vi "NXTMMX-DM.old2.vi"(0 "Input of Motor Multiplexer":T4={"NXTMMX Address"=6, "Which Motor"=0, "Operation"=0, "Next Action"=0, "Position"=0, "Direction"=FALSE, "Power"=100, "Durartion"=0, "Wait for Completion"=FALSE, "Relative"=FALSE, "PID"={"Write PID"=FALSE, "PKp"=100, "PKi"=100, "PKd"=100, "SKp "=100, "SKi"=100, "SKd"=100, "passcount"=0, "tolerance"=0}} {"Next Action" items=["Float", "Brake"]; "Operation" items=["Run Unlimited", "Run Seconds", "Run Tachometer"]; "Which Motor" items=["Motor 1", "Motor 2", "Both Motors"]; "NXTMMX Address" min=2 max=254 step=2 format="%x"}, 2 "NXT":T2={"Hardware"="NXT", "Flattened String"=""}, 3 "Input Port":T3 items=["Port 1", "Port 2", "Port 3", "Port 4"]) -> (1 "Output of Motor Multiplexer":T1, 4 "NXT dup":T2={"Hardware"="NXT", "Flattened String"=""})   [LabVIEW 2010]
uses:
  <vilib>/NXT/Block Support/NXT_InputPort.ctl
  <vilib>/NXT/Subs/LVHSConnector.ctl
  <vilib>/NXT/Block Support/HWPage.SensorType.ctl
  <vilib>/NXT/Block Support/HWPage.SensorMode.ctl
  <vilib>/NXT/Dual Mode Library/Waits/Wait_Num(msec).vi
panel:
  out "Address":i32
  # "mindsensors.com\nCopyright (c) 2009 by mindsensors.com\nEmail: info (<at>) mindsensors (<dot>) com\n\nThis program is free software. You can redistribute it and/or modify\nit under the terms of the GNU General Public License as published by\nthe Free Software Foundation; version 3 of the License.\nRead the license at: http://www.gnu.org/licenses/gpl.txt"
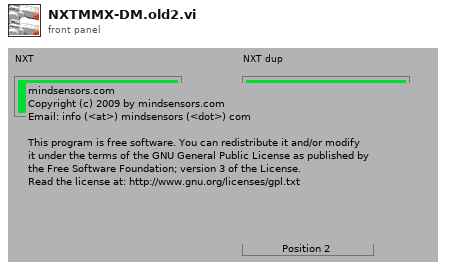
[diagram p1: front panel]
types:
  T1 = cluster{"Milivolts":u16, "Position 1":i32, "Position 2":i32, "Motor battery Voltage":dbl}
  T2 = typedef "LVHSConnector.ctl" = cluster{"Hardware":string, "Flattened String":string}
  T3 = typedef "NXT_InputPort.ctl" = u8
  T4 = cluster{"NXTMMX Address":u8, "Which Motor":u8, "Operation":u8, "Next Action":u8, "Position":i32, "Direction":bool, "Power":i8, "Durartion":u8, "Wait for Completion":bool, "Relative":bool, "PID":cluster{"Write PID":bool, "PKp":u16, "PKi":u16, "PKd":u16, "SKp ":u16, "SKi":u16, "SKd":u16, "passcount":u8, "tolerance":u8}}
  T5 = typedef "HWPage.SensorType.ctl" = u8
  T6 = typedef "HWPage.SensorMode.ctl" = u8
  T7 = cluster{"Write PID":bool, "PKp":u16, "PKi":u16, "PKd":u16, "SKp ":u16, "SKi":u16, "SKd":u16, "passcount":u8, "tolerance":u8}
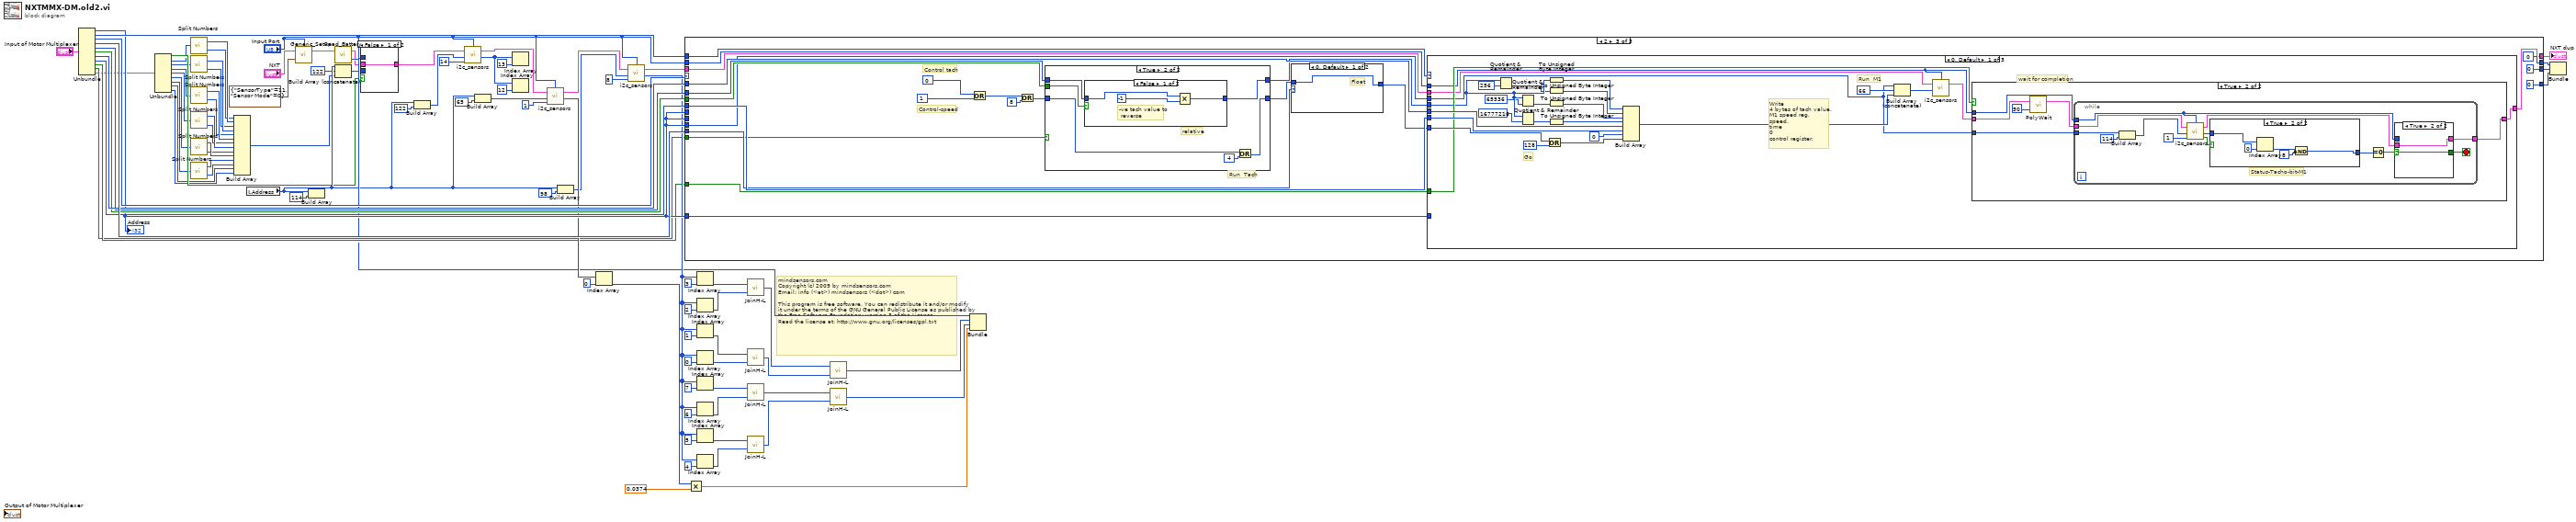
[diagram p0: block diagram]
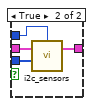
[diagram p2: hidden frame]
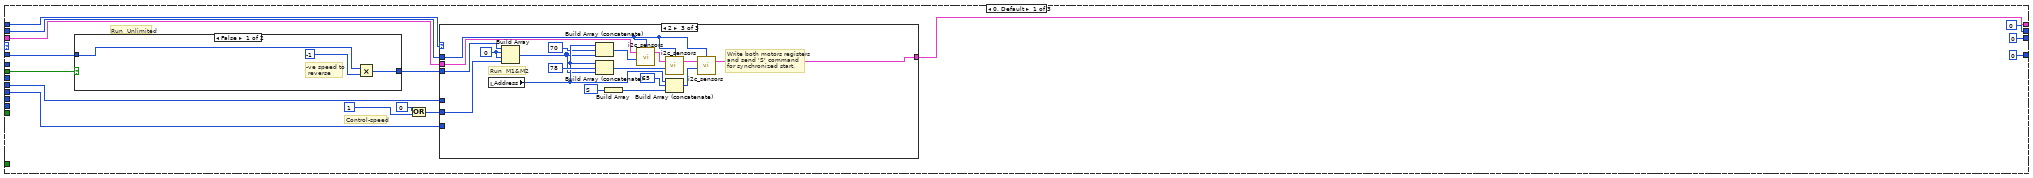
[diagram p3: hidden frame]
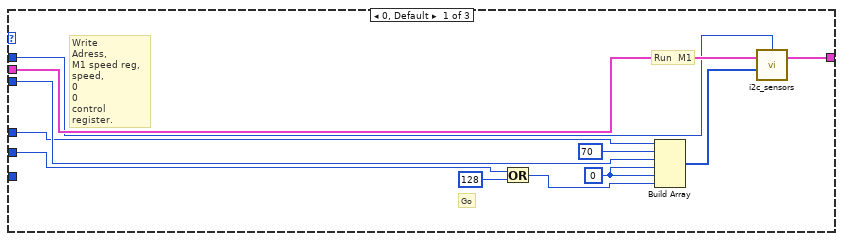
[diagram p4: hidden frame]
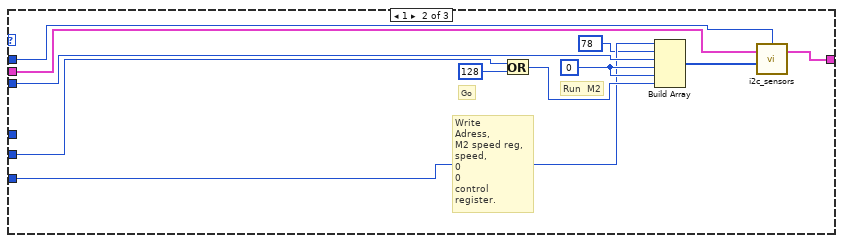
[diagram p5: hidden frame]
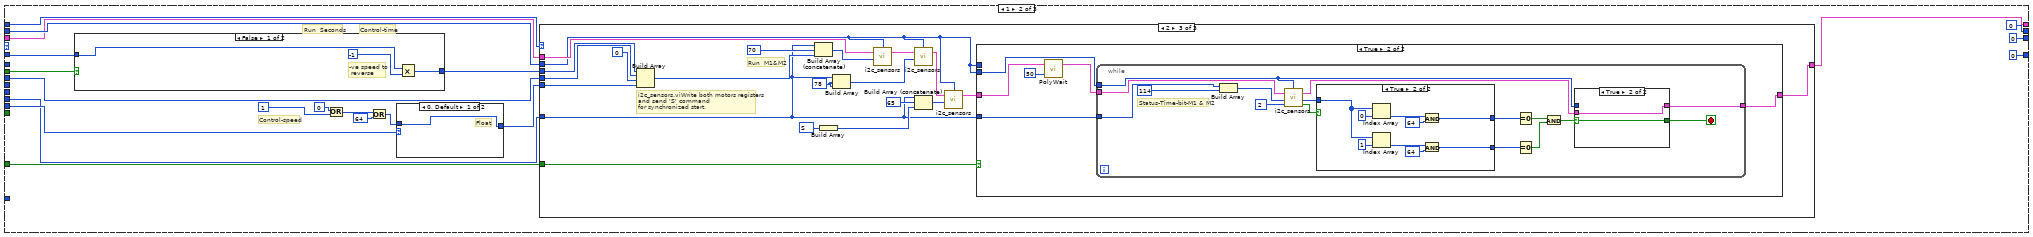
[diagram p7: hidden frame]
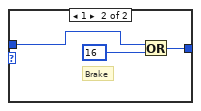
[diagram p8: hidden frame]
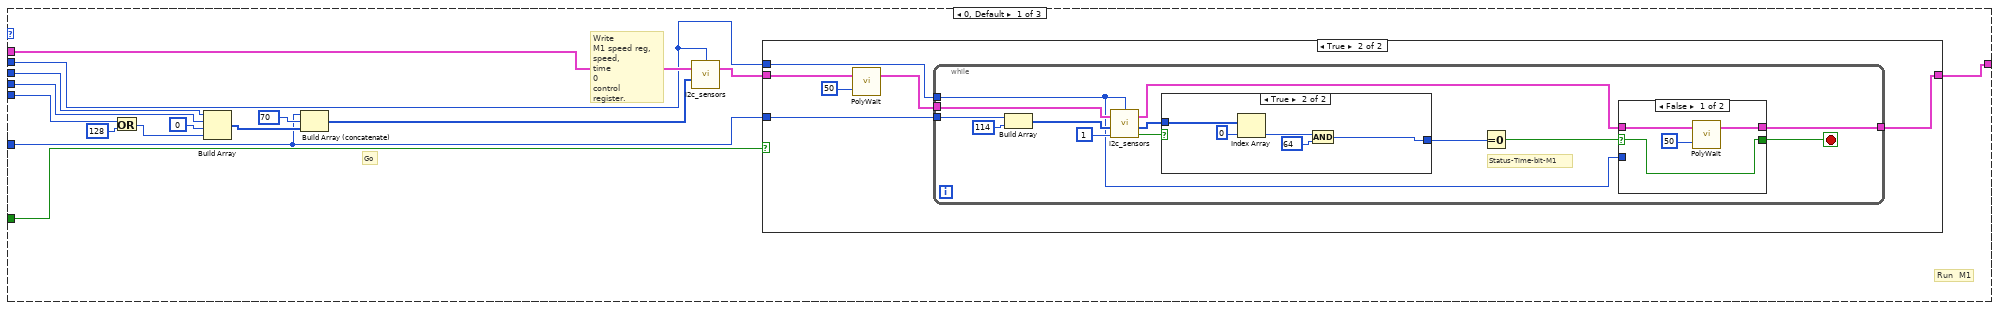
[diagram p9: hidden frame]
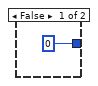
[diagram p12: hidden frame]
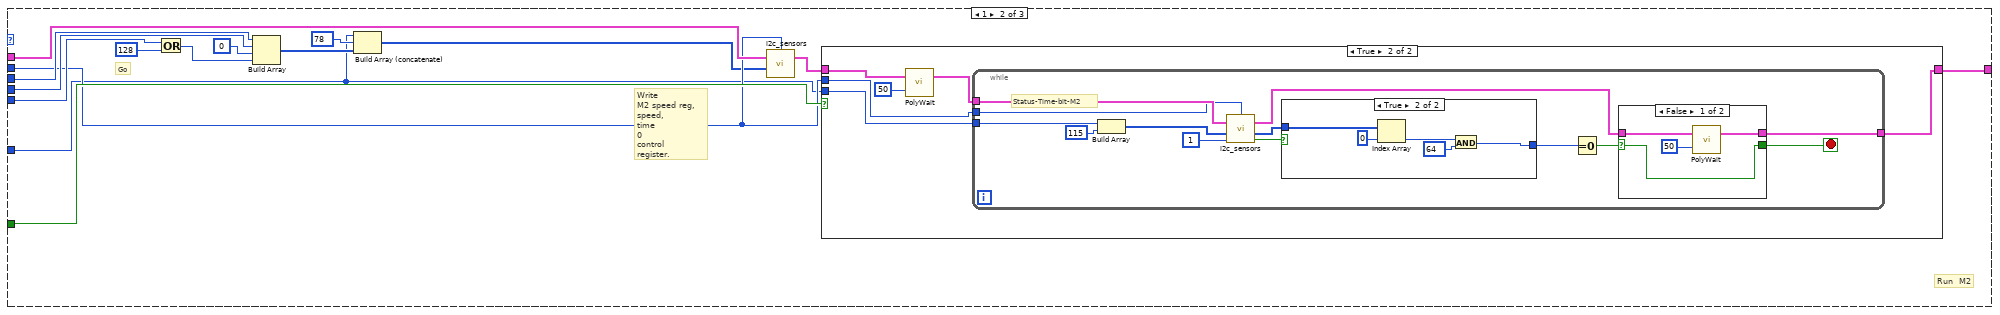
[diagram p13: hidden frame]
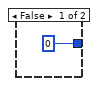
[diagram p16: hidden frame]
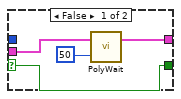
[diagram p18: hidden frame]
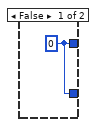
[diagram p19: hidden frame]
diagram:
  # "mindsensors.com\nCopyright (c) 2009 by mindsensors.com\nEmail: info (<at>) mindsensors (<dot>) com\n\nThis program is free software. You can redistribute it and/or modify\nit under the terms of the GNU General Public License as published by\nthe Free Software Foundation; version 3 of the License.\nRead the license at: http://www.gnu.org/licenses/gpl.txt"
  n1 = Unbundle("Input of Motor Multiplexer") -> ("NXTMMX Address"=w84:u8, "Which Motor"=w86:u8, "Operation"=w91:u8, "Next Action"=w90:u8, "Position"=w88:i32, "Direction"=w87:bool, "Power"=w89:i8, "Durartion"=w85:u8, "Wait for Completion"=w50:bool, "Relative"=w49:bool, "PID"=w33:T7)
  "Address" <- w84
  n2 = Unbundle(w33) -> ("Write PID"=w36:bool, "PKp"=w18:u16, "PKi"=w15:u16, "PKd"=w10:u16, "SKp"=w7:u16, "SKi"=w4:u16, "SKd"=w3:u16, "passcount"=w35:u8, "tolerance"=w34:u8)
  n3 = call <vilib>:"Split Numbers.vi"("(hi.lo)"=w18) -> ("low"=w16:u8, "hi"=w17:u8)
  n4 = call <vilib>:"Split Numbers.vi"("(hi.lo)"=w15) -> ("low"=w13:u8, "hi"=w14:u8)
  n5 = call <vilib>:"Split Numbers.vi"("(hi.lo)"=w10) -> ("low"=w11:u8, "hi"=w12:u8)
  n6 = call <vilib>:"Split Numbers.vi"("(hi.lo)"=w7) -> ("low"=w8:u8, "hi"=w9:u8)
  n7 = call <vilib>:"Split Numbers.vi"("(hi.lo)"=w4) -> ("low"=w5:u8, "hi"=w6:u8)
  n8 = call <vilib>:"Split Numbers.vi"("(hi.lo)"=w3) -> ("low"=w1:u8, "hi"=w2:u8)
  n9 = Build Array(w16, w17, w13, w14, w11, w12, w8, w9, w5, w6, w2, w1, w35, w34) -> (w41:u8[])
  n10 = local read "Address"() -> (w43:i32)
  n11 = call <vilib>:"Generic_Setup.vi"("Sensor Setup"=cluster{"SensorType":T5, "Sensor Mode":T6} {"SensorType"=11, "Sensor Mode"=0}, "NXT"="NXT", "Port"="Input Port") -> ("NXT"=w82:T2)  [unwired: 1 out]
  n12 = Build Array(w43, u8 114 ("Reg Address")) -> ()  [unwired: 1 out]
  n13 = call <vilib>:"Read_Battery.vi"("NXT"=w82) -> ("millivolts"=w48:i32, "NXT"=w38:T2)  [unwired: 2 in]
  n14 = Build Array (concatenate)(w43, u8 122 ("Reg Address"), w41) -> (w40:i32[])
  n15 = case shown="False" w36 {
    tunnel: w40 -> [_ w97]
    tunnel: "Input Port" -> [_ w96]
    tunnel: w38 -> [w93 w95]
    tunnel: [w93 w94] -> w37
    frame False {
    }
    frame True {
      n16 = call <vilib>:"i2c_sensors.vi"("Bytes to Write"=w97, "NXT"=w95, "Port"=w96) -> ("NXT"=w94:T2)  [unwired: 2 in, 2 out]
    }
  }
  n17 = Build Array(w43, u8 122 ("Reg Address")) -> (w67:i32[])
  n18 = call <vilib>:"i2c_sensors.vi"("Return Length"=u8 14 ("bytes to read"), "Bytes to Write"=w67, "NXT"=w37, "Port"="Input Port") -> ("Bytes read"=w65:u8[], "NXT"=w60:T2)  [unwired: 1 in, 1 out]
  n19 = Build Array(w43, u8 65 ("Reg Address")) -> (w62:i32[])
  n20 = Index Array(array=w65, index=13) -> ()  [unwired: 1 out]
  n21 = Index Array(array=w65, index=12) -> ()  [unwired: 1 out]
  n22 = call <vilib>:"i2c_sensors.vi"("Return Length"=u8 1 ("bytes to read"), "Bytes to Write"=w62, "NXT"=w60, "Port"="Input Port") -> ("Bytes read"=w61:u8[], "NXT"=w55:T2)  [unwired: 1 in, 1 out]
  n23 = Build Array(w43, u8 98 ("Reg Address")) -> (w59:i32[])
  n24 = Index Array(array=w61, index=0) -> (element=w70:u8)
  n25 = call <vilib>:"i2c_sensors.vi"("Return Length"=u8 8 ("bytes to read"), "Bytes to Write"=w59, "NXT"=w55, "Port"="Input Port") -> ("Bytes read"=w56:u8[], "NXT"=w52:T2)  [unwired: 1 in, 1 out]
  n26 = case shown="2" w91 {
    tunnel: w87 -> [w110 w174 w360]
    tunnel: w89 -> [w109 w173 w350]
    tunnel: w86 -> [w108 w172 w359]
    tunnel: "Input Port" -> [w106 w170 w358]
    tunnel: w85 -> [_ w167 w355]
    tunnel: w90 -> [_ w166 w354]
    tunnel: w88 -> [_ _ w351]
    tunnel: w50 -> [_ w163 w352]
    tunnel: w49 -> [_ _ w348]
    tunnel: [0 0 0] -> w47
    tunnel: [u32 0 ("Out") u32 0 ("Out") u32 0 ("Out")] -> w46
    tunnel: [u16 0 u16 0 u16 0] -> w45
    tunnel: w52 -> [w101 w159 w341]
    tunnel: [w100 w158 w342] -> w44
    tunnel: w84 -> [_ w157 w340]
    tunnel: w84 -> [w99 _ _]
    tunnel: w84 -> [_ _ w339]
    tunnel: w84 -> [w98 _ _]
    frame 0, Default {
      # "Control-speed"
      # "Run  Unlimited"
      n27 = case shown="False" w110 {
        tunnel: w109 -> [w155 w156]
        tunnel: [w153 w156] -> w107
        frame False {
          # "-ve speed to\n reverse"
          n28 = Multiply(x=w155, y=i8 -1) -> (x*y=w153:i8)
        }
        frame True {
        }
      }
      n29 = Or(x=0, y=1) -> (x .or. y?=w105:i32)
      n30 = case shown="2" w108 {
        tunnel: w105 -> [w122 w133 w149]
        tunnel: w107 -> [w121 w132 w152]
        tunnel: w106 -> [w116 w129 w144]
        tunnel: w101 -> [w118 w128 w148]
        tunnel: [w117 w127 w139] -> w100
        tunnel: w99 -> [w115 _ _]
        tunnel: w98 -> [_ w126 _]
        frame 0, Default {
          w120 = 0
          # "Go"
          # "Run  M1"
          # "Write \nAdress,\nM1 speed reg,\nspeed,\n0\n0\ncontrol register."
          n31 = Or(x=w122, y=128) -> (x .or. y?=w119:i32)
          n32 = Build Array(w115, 70, w121, w120, w120, w119) -> (w113:i32[])
          n33 = call <vilib>:"i2c_sensors.vi"("Bytes to Write"=w113, "NXT"=w118, "Port"=w116) -> ("NXT"=w117:T2)  [unwired: 2 in, 2 out]
        }
        frame 1 {
          w131 = 0
          # "Go"
          # "Run  M2"
          # "Write\nAdress, \nM2 speed reg,\nspeed,\n0\n0\ncontrol register."
          n34 = Or(x=w133, y=128) -> (x .or. y?=w130:i32)
          n35 = Build Array(w126, 78, w132, w131, w131, w130) -> (w124:i32[])
          n36 = call <vilib>:"i2c_sensors.vi"("Bytes to Write"=w124, "NXT"=w128, "Port"=w129) -> ("NXT"=w127:T2)  [unwired: 2 in, 2 out]
        }
        frame 2 {
          w150 = u16 83 items=["S"=83]
          w151 = 0
          # "Write both motors registers\nand send 'S' command \nfor synchronized start."
          # "Run  M1&M2"
          n37 = local read "Address"() -> (w138:i32)
          n38 = Build Array(w152, w151, w151, w149) -> (w135:i32[])
          n39 = Build Array (concatenate)(w138, 70, w135) -> (w136:i32[])
          n40 = Build Array (concatenate)(w138, 78, w135) -> (w146:i32[])
          n41 = Build Array(w150) -> (w142:u16[])
          n42 = call <vilib>:"i2c_sensors.vi"("Bytes to Write"=w136, "NXT"=w148, "Port"=w144) -> ("NXT"=w145:T2)  [unwired: 2 in, 2 out]
          n43 = call <vilib>:"i2c_sensors.vi"("Bytes to Write"=w146, "NXT"=w145, "Port"=w144) -> ("NXT"=w143:T2)  [unwired: 2 in, 2 out]
          n44 = Build Array (concatenate)(w138, 65, w142) -> (w140:i32[])
          n45 = call <vilib>:"i2c_sensors.vi"("Bytes to Write"=w140, "NXT"=w143, "Port"=w144) -> ("NXT"=w139:T2)  [unwired: 2 in, 2 out]
        }
      }
    }
    frame 1 {
      # "Control-time"
      # "Control-speed"
      # "Run  Seconds"
      n46 = case shown="False" w174 {
        tunnel: w173 -> [w337 w338]
        tunnel: [w335 w338] -> w171
        frame False {
          # "-ve speed to\n reverse"
          n47 = Multiply(x=w337, y=i8 -1) -> (x*y=w335:i8)
        }
        frame True {
        }
      }
      n48 = Or(x=0, y=1) -> (x .or. y?=w168:i32)
      n49 = Or(x=w168, y=64) -> (x .or. y?=w165:i32)
      n50 = case shown="0, Default" w166 {
        tunnel: w165 -> [w177 w179]
        tunnel: [w177 w180] -> w164
        frame 0, Default {
          # "Float"
        }
        frame 1 {
          # "Brake"
          n51 = Or(x=w179, y=16) -> (x .or. y?=w180:i32)
        }
      }
      n52 = case shown="2" w172 {
        tunnel: w164 -> [w194 w241 w292]
        tunnel: w171 -> [w193 w240 w295]
        tunnel: w170 -> [w183 w232 w277]
        tunnel: w167 -> [w190 w237 w291]
        tunnel: w163 -> [w189 w236 w290]
        tunnel: w159 -> [w187 w235 w286]
        tunnel: [w182 w229 w276] -> w158
        tunnel: w157 -> [w181 w228 w275]
        frame 0, Default {
          # "Go"
          # "Run  M1"
          # "Write \nM1 speed reg,\nspeed,\ntime\n0\ncontrol register."
          n53 = Or(x=w194, y=128) -> (x .or. y?=w191:i32)
          n54 = Build Array(w193, w190, 0, w191) -> (w184:i32[])
          n55 = Build Array (concatenate)(w181, 70, w184) -> (w186:i32[])
          n56 = call <vilib>:"i2c_sensors.vi"("Bytes to Write"=w186, "NXT"=w187, "Port"=w183) -> ("NXT"=w188:T2)  [unwired: 2 in, 2 out]
          n57 = case shown="True" w189 {
            tunnel: w183 -> [_ w202]
            tunnel: w188 -> [w196 w200]
            tunnel: [w196 w198] -> w182
            tunnel: w181 -> [_ w197]
            frame False {
            }
            frame True {
              n58 = call-poly <vilib>:"PolyWait.vi"("Time (100 msec)"=u16 50 ("Delay ms"), "NXT"=w200) -> ("NXT"=w199:T2)  [unwired: 2 in]
              n59 = while {
                tunnel: w202 -> [w206]
                tunnel: w199 -> [w211]
                tunnel: [w210] -> w198
                tunnel: w197 -> [w204]
                stop <- w214 stop-if-true
                # "Status-Time-bit-M1"
                n60 = Build Array(w204, 114) -> (w207:i32[])
                n61 = call <vilib>:"i2c_sensors.vi"("Return Length"=1, "Bytes to Write"=w207, "NXT"=w211, "Port"=w206) -> ("Success?"=w203:bool, "Bytes read"=w209:u8[], "NXT"=w212:T2)  [unwired: 1 in]
                n62 = case shown="True" w203 {
                  tunnel: w209 -> [_ w227]
                  tunnel: [u8 0 w223] -> w215
                  frame False {
                  }
                  frame True {
                    n63 = Index Array(array=w227, index=0) -> (element=w224:u8)
                    n64 = And(x=w224, y=u8 64) -> (x .and. y?=w223:u8)
                  }
                }
                n65 = Equal To 0?(x=w215) -> (x = 0?=w213:bool)
                n66 = case shown="False" w213 {
                  selector: w213 -> [w219 w221]
                  tunnel: w206 -> [_ _]
                  tunnel: [w219 w221] -> w214
                  tunnel: w212 -> [w217 w220]
                  tunnel: [w216 w220] -> w210
                  frame False {
                    n67 = call-poly <vilib>:"PolyWait.vi"("Time (100 msec)"=u16 50 ("Delay ms"), "NXT"=w217) -> ("NXT"=w216:T2)  [unwired: 2 in]
                  }
                  frame True {
                  }
                }
              }
            }
          }
        }
        frame 1 {
          # "Go"
          # "Run  M2"
          # "Write \nM2 speed reg,\nspeed,\ntime\n0\ncontrol register."
          n68 = Or(x=w241, y=128) -> (x .or. y?=w238:i32)
          n69 = Build Array(w240, w237, 0, w238) -> (w233:i32[])
          n70 = Build Array (concatenate)(w228, 78, w233) -> (w231:i32[])
          n71 = call <vilib>:"i2c_sensors.vi"("Bytes to Write"=w231, "NXT"=w235, "Port"=w232) -> ("NXT"=w230:T2)  [unwired: 2 in, 2 out]
          n72 = case shown="True" w236 {
            tunnel: w232 -> [_ w249]
            tunnel: w230 -> [w243 w247]
            tunnel: [w243 w245] -> w229
            tunnel: w228 -> [_ w244]
            frame False {
            }
            frame True {
              n73 = call-poly <vilib>:"PolyWait.vi"("Time (100 msec)"=u16 50 ("Delay ms"), "NXT"=w247) -> ("NXT"=w246:T2)  [unwired: 2 in]
              n74 = while {
                tunnel: w249 -> [w256]
                tunnel: w246 -> [w257]
                tunnel: [w259] -> w245
                tunnel: w244 -> [w251]
                stop <- w261 stop-if-true
                # "Status-Time-bit-M2"
                n75 = Build Array(w251, 115) -> (w253:i32[])
                n76 = call <vilib>:"i2c_sensors.vi"("Return Length"=1, "Bytes to Write"=w253, "NXT"=w257, "Port"=w256) -> ("Success?"=w250:bool, "Bytes read"=w252:u8[], "NXT"=w258:T2)  [unwired: 1 in]
                n77 = case shown="True" w250 {
                  tunnel: w252 -> [_ w274]
                  tunnel: [u8 0 w270] -> w262
                  frame False {
                  }
                  frame True {
                    n78 = Index Array(array=w274, index=0) -> (element=w271:u8)
                    n79 = And(x=w271, y=u8 64) -> (x .and. y?=w270:u8)
                  }
                }
                n80 = Equal To 0?(x=w262) -> (x = 0?=w260:bool)
                n81 = case shown="False" w260 {
                  selector: w260 -> [w266 w268]
                  tunnel: [w266 w268] -> w261
                  tunnel: [w264 w267] -> w259
                  tunnel: w258 -> [w263 w267]
                  frame False {
                    n82 = call-poly <vilib>:"PolyWait.vi"("Time (100 msec)"=u16 50 ("Delay ms"), "NXT"=w263) -> ("NXT"=w264:T2)  [unwired: 2 in]
                  }
                  frame True {
                  }
                }
              }
            }
          }
        }
        frame 2 {
          w293 = u16 83 items=["S"=83]
          w285 = 78
          # "i2c_sensors.viWrite both motors registers\nand send 'S' command \nfor synchronized start."
          # "Run  M1&M2"
          n83 = Build Array(w295, w291, 0, w292) -> (w288:i32[])
          n84 = Build Array (concatenate)(w275, 70, w288) -> (w287:i32[])
          n85 = Build Array(w293) -> (w283:u16[])
          n86 = Build Array(w275, w285, w285) -> (w280:i32[])
          n87 = call <vilib>:"i2c_sensors.vi"("Bytes to Write"=w287, "NXT"=w286, "Port"=w277) -> ("NXT"=w281:T2)  [unwired: 2 in, 2 out]
          n88 = call <vilib>:"i2c_sensors.vi"("Bytes to Write"=w280, "NXT"=w281, "Port"=w277) -> ("NXT"=w282:T2)  [unwired: 2 in, 2 out]
          n89 = Build Array (concatenate)(w275, 65, w283) -> (w279:i32[])
          n90 = call <vilib>:"i2c_sensors.vi"("Bytes to Write"=w279, "NXT"=w282, "Port"=w277) -> ("NXT"=w278:T2)  [unwired: 2 in, 2 out]
          n91 = case shown="True" w290 {
            tunnel: w277 -> [_ _]
            tunnel: w278 -> [w296 w301]
            tunnel: w277 -> [_ w299]
            tunnel: [w296 w298] -> w276
            tunnel: w275 -> [_ w297]
            frame False {
            }
            frame True {
              n92 = call-poly <vilib>:"PolyWait.vi"("Time (100 msec)"=u16 50 ("Delay ms"), "NXT"=w301) -> ("NXT"=w300:T2)  [unwired: 2 in]
              n93 = while {
                tunnel: w300 -> [w306]
                tunnel: w299 -> [w309]
                tunnel: [w305] -> w298
                tunnel: w297 -> [w304]
                stop <- w313 stop-if-true
                # "Status-Time-bit-M1 & M2"
                n94 = Build Array(w304, 114) -> (w310:i32[])
                n95 = call <vilib>:"i2c_sensors.vi"("Return Length"=2, "Bytes to Write"=w310, "NXT"=w306, "Port"=w309) -> ("Success?"=w303:bool, "Bytes read"=w308:u8[], "NXT"=w307:T2)  [unwired: 1 in]
                n96 = case shown="True" w303 {
                  tunnel: w308 -> [_ w333]
                  tunnel: [w325 w326] -> w318
                  tunnel: [w325 w328] -> w317
                  frame False {
                    w325 = u8 0
                  }
                  frame True {
                    n97 = Index Array(array=w333, index=0) -> (element=w329:u8)
                    n98 = Index Array(array=w333, index=1) -> (element=w327:u8)
                    n99 = And(x=w329, y=u8 64) -> (x .and. y?=w328:u8)
                    n100 = And(x=w327, y=u8 64) -> (x .and. y?=w326:u8)
                  }
                }
                n101 = Equal To 0?(x=w317) -> (x = 0?=w316:bool)
                n102 = Equal To 0?(x=w318) -> (x = 0?=w315:bool)
                n103 = And(x=w316, y=w315) -> (x .and. y?=w314:bool)
                n104 = case shown="True" w314 {
                  selector: w314 -> [w322 w324]
                  tunnel: w309 -> [_ _]
                  tunnel: [w322 w324] -> w313
                  tunnel: w307 -> [w320 w323]
                  tunnel: [w319 w323] -> w305
                  frame False {
                    n105 = call-poly <vilib>:"PolyWait.vi"("Time (100 msec)"=u16 50 ("Delay ms"), "NXT"=w320) -> ("NXT"=w319:T2)  [unwired: 2 in]
                  }
                  frame True {
                  }
                }
              }
            }
          }
        }
      }
    }
    frame 2 {
      # "Run  Tach"
      # "Control tach"
      # "Control-speed"
      n106 = Or(x=0, y=1) -> (x .or. y?=w356:i32)
      n107 = Or(x=w356, y=8) -> (x .or. y?=w347:i32)
      n108 = case shown="True" w348 {
        tunnel: w360 -> [_ w370]
        tunnel: w351 -> [w364 w369]
        tunnel: [w364 w368] -> w349
        tunnel: w347 -> [w363 w367]
        tunnel: [w363 w365] -> w346
        frame False {
          # "absolute\nignore the direction"
        }
        frame True {
          # "relative"
          n109 = case shown="False" w370 {
            tunnel: w369 -> [w373 w374]
            tunnel: [w371 w374] -> w368
            frame False {
              # "-ve tach value to\n reverse"
              n110 = Multiply(x=w373, y=i8 -1) -> (x*y=w371:i32)
            }
            frame True {
            }
          }
          n111 = Or(x=w367, y=4) -> (x .or. y?=w365:i32)
        }
      }
      n112 = case shown="0, Default" w354 {
        tunnel: [w375 w378] -> w353
        tunnel: w346 -> [w375 w376]
        frame 0, Default {
          # "Float"
        }
        frame 1 {
          # "Brake"
          n113 = Or(x=w376, y=16) -> (x .or. y?=w378:i32)
        }
      }
      n114 = case shown="0, Default" w359 {
        tunnel: w353 -> [w403 w461 w524]
        tunnel: w358 -> [w385 w442 w496]
        tunnel: w355 -> [w399 w457 w523]
        tunnel: w352 -> [w398 w456 w522]
        tunnel: w350 -> [w402 w460 w521]
        tunnel: w349 -> [w396 w449 w514]
        tunnel: [w379 w437 w509] -> w342
        tunnel: w341 -> [w382 w440 w508]
        tunnel: w340 -> [w380 _ _]
        tunnel: w339 -> [_ w438 _]
        frame 0, Default {
          # "wait for completion"
          # "Go"
          # "Run  M1"
          # "Write\n4 bytes of tach value. \nM1 speed reg,\nspeed,\ntime\n0\ncontrol register."
          n115 = Quotient & Remainder(x=w396, y=u32 256) -> (floor(x/y)=w392:u32)  [unwired: 1 out]
          n116 = Quotient & Remainder(x=w396, y=u32 65536) -> (floor(x/y)=w390:u32)  [unwired: 1 out]
          n117 = Quotient & Remainder(x=w396, y=u32 16777216) -> (floor(x/y)=w387:u32)  [unwired: 1 out]
          n118 = Or(x=w403, y=128) -> (x .or. y?=w400:i32)
          n119 = To Unsigned Byte Integer(number=w396) -> (unsigned 8bit integer=w397:u8)
          n120 = To Unsigned Byte Integer(number=w392) -> (unsigned 8bit integer=w391:u8)
          n121 = To Unsigned Byte Integer(number=w390) -> (unsigned 8bit integer=w389:u8)
          n122 = To Unsigned Byte Integer(number=w387) -> (unsigned 8bit integer=w388:u8)
          n123 = Build Array(w397, w391, w389, w388, w402, w399, 0, w400) -> (w386:i32[])
          n124 = Build Array (concatenate)(w380, 66, w386) -> (w383:i32[])
          n125 = call <vilib>:"i2c_sensors.vi"("Bytes to Write"=w383, "NXT"=w382, "Port"=w385) -> ("NXT"=w381:T2)  [unwired: 2 in, 2 out]
          n126 = case shown="True" w398 {
            tunnel: w385 -> [_ w411]
            tunnel: w381 -> [w405 w409]
            tunnel: w380 -> [_ w408]
            tunnel: [w405 w406] -> w379
            frame False {
            }
            frame True {
              n127 = call-poly <vilib>:"PolyWait.vi"("Time (100 msec)"=u16 50 ("Delay ms"), "NXT"=w409) -> ("NXT"=w407:T2)  [unwired: 2 in]
              n128 = while {
                tunnel: w411 -> [w419]
                tunnel: w408 -> [w417]
                tunnel: w407 -> [w416]
                tunnel: [w414] -> w406
                stop <- w422 stop-if-true
                # "Status-Tacho-bit-M1"
                n129 = Build Array(w417, 114) -> (w412:i32[])
                n130 = call <vilib>:"i2c_sensors.vi"("Return Length"=1, "Bytes to Write"=w412, "NXT"=w416, "Port"=w419) -> ("Success?"=w413:bool, "Bytes read"=w420:u8[], "NXT"=w415:T2)  [unwired: 1 in]
                n131 = case shown="True" w413 {
                  tunnel: w420 -> [_ w436]
                  tunnel: [u8 0 w432] -> w424
                  frame False {
                  }
                  frame True {
                    n132 = Index Array(array=w436, index=0) -> (element=w433:u8)
                    n133 = And(x=w433, y=u8 8) -> (x .and. y?=w432:u8)
                  }
                }
                n134 = Equal To 0?(x=w424) -> (x = 0?=w423:bool)
                n135 = case shown="True" w423 {
                  selector: w423 -> [w428 w430]
                  tunnel: w419 -> [_ _]
                  tunnel: [w428 w430] -> w422
                  tunnel: w415 -> [w426 w429]
                  tunnel: [w425 w429] -> w414
                  frame False {
                    n136 = call-poly <vilib>:"PolyWait.vi"("Time (100 msec)"=u16 50 ("Delay ms"), "NXT"=w426) -> ("NXT"=w425:T2)  [unwired: 2 in]
                  }
                  frame True {
                  }
                }
              }
            }
          }
        }
        frame 1 {
          # "Go"
          # "Run  M2"
          # "Write \nM2 speed reg,\nspeed,\ntime\n0\ncontrol register."
          n137 = Quotient & Remainder(x=w449, y=u32 256) -> (floor(x/y)=w452:u32)  [unwired: 1 out]
          n138 = Quotient & Remainder(x=w449, y=u32 65536) -> (floor(x/y)=w451:u32)  [unwired: 1 out]
          n139 = Quotient & Remainder(x=w449, y=u32 16777216) -> (floor(x/y)=w450:u32)  [unwired: 1 out]
          n140 = Or(x=w461, y=128) -> (x .or. y?=w458:i32)
          n141 = To Unsigned Byte Integer(number=w449) -> (unsigned 8bit integer=w448:u8)
          n142 = To Unsigned Byte Integer(number=w452) -> (unsigned 8bit integer=w447:u8)
          n143 = To Unsigned Byte Integer(number=w451) -> (unsigned 8bit integer=w446:u8)
          n144 = To Unsigned Byte Integer(number=w450) -> (unsigned 8bit integer=w445:u8)
          n145 = Build Array(w448, w447, w446, w445, w460, w457, 0, w458) -> (w443:i32[])
          n146 = Build Array (concatenate)(w438, 74, w443) -> (w441:i32[])
          n147 = call <vilib>:"i2c_sensors.vi"("Bytes to Write"=w441, "NXT"=w440, "Port"=w442) -> ("NXT"=w439:T2)  [unwired: 2 in, 2 out]
          n148 = case shown="True" w456 {
            tunnel: w442 -> [_ w469]
            tunnel: w439 -> [w463 w467]
            tunnel: w438 -> [_ w465]
            tunnel: [w463 w464] -> w437
            frame False {
            }
            frame True {
              n149 = call-poly <vilib>:"PolyWait.vi"("Time (100 msec)"=u16 50 ("Delay ms"), "NXT"=w467) -> ("NXT"=w466:T2)  [unwired: 2 in]
              n150 = while {
                tunnel: w469 -> [w473]
                tunnel: w466 -> [w479]
                tunnel: w465 -> [w477]
                tunnel: [w470] -> w464
                stop <- w480 stop-if-true
                # "Status-Tacho-bit-M2"
                n151 = Build Array(w477, 115) -> (w475:i32[])
                n152 = call <vilib>:"i2c_sensors.vi"("Return Length"=1, "Bytes to Write"=w475, "NXT"=w479, "Port"=w473) -> ("Success?"=w472:bool, "Bytes read"=w474:u8[], "NXT"=w471:T2)  [unwired: 1 in]
                n153 = case shown="True" w472 {
                  tunnel: w474 -> [_ w494]
                  tunnel: [u8 0 w490] -> w482
                  frame False {
                  }
                  frame True {
                    n154 = Index Array(array=w494, index=0) -> (element=w492:u8)
                    n155 = And(x=w492, y=u8 8) -> (x .and. y?=w490:u8)
                  }
                }
                n156 = Equal To 0?(x=w482) -> (x = 0?=w481:bool)
                n157 = case shown="True" w481 {
                  selector: w481 -> [w486 w488]
                  tunnel: w473 -> [_ _]
                  tunnel: [w486 w488] -> w480
                  tunnel: w471 -> [w484 w487]
                  tunnel: [w483 w487] -> w470
                  frame False {
                    n158 = call-poly <vilib>:"PolyWait.vi"("Time (100 msec)"=u16 50 ("Delay ms"), "NXT"=w484) -> ("NXT"=w483:T2)  [unwired: 2 in]
                  }
                  frame True {
                  }
                }
              }
            }
          }
        }
        frame 2 {
          w525 = u16 83 items=["S"=83]
          # "Write both motors registers\nand send 'S' command \nfor synchronized start."
          # "Run  M1&M2"
          n159 = Quotient & Remainder(x=w514, y=u32 256) -> (floor(x/y)=w517:u32)  [unwired: 1 out]
          n160 = Quotient & Remainder(x=w514, y=u32 65536) -> (floor(x/y)=w516:u32)  [unwired: 1 out]
          n161 = Quotient & Remainder(x=w514, y=u32 16777216) -> (floor(x/y)=w515:u32)  [unwired: 1 out]
          n162 = To Unsigned Byte Integer(number=w514) -> (unsigned 8bit integer=w513:u8)
          n163 = To Unsigned Byte Integer(number=w517) -> (unsigned 8bit integer=w512:u8)
          n164 = To Unsigned Byte Integer(number=w516) -> (unsigned 8bit integer=w511:u8)
          n165 = To Unsigned Byte Integer(number=w515) -> (unsigned 8bit integer=w510:u8)
          n166 = local read "Address"() -> (w495:i32)
          n167 = Build Array(w513, w512, w511, w510, w521, w523, 0, w524) -> (w499:i32[])
          n168 = Build Array (concatenate)(w495, 74, w499) -> (w504:i32[])
          n169 = Build Array (concatenate)(w495, 66, w499) -> (w502:i32[])
          n170 = Build Array(w525) -> (w497:u16[])
          n171 = call <vilib>:"i2c_sensors.vi"("Bytes to Write"=w502, "NXT"=w508, "Port"=w496) -> ("NXT"=w505:T2)  [unwired: 2 in, 2 out]
          n172 = call <vilib>:"i2c_sensors.vi"("Bytes to Write"=w504, "NXT"=w505, "Port"=w496) -> ("NXT"=w506:T2)  [unwired: 2 in, 2 out]
          n173 = Build Array (concatenate)(w495, 65, w497) -> (w503:i32[])
          n174 = call <vilib>:"i2c_sensors.vi"("Bytes to Write"=w503, "NXT"=w506, "Port"=w496) -> ("NXT"=w507:T2)  [unwired: 2 in, 2 out]
          n175 = case shown="True" w522 {
            tunnel: w496 -> [_ w533]
            tunnel: w507 -> [w527 w531]
            tunnel: [w527 w530] -> w509
            tunnel: w495 -> [_ w528]
            frame False {
            }
            frame True {
              n176 = call-poly <vilib>:"PolyWait.vi"("Time (100 msec)"=u16 50 ("Delay ms"), "NXT"=w531) -> ("NXT"=w529:T2)  [unwired: 2 in]
              n177 = while {
                tunnel: w533 -> [w538]
                tunnel: [w543] -> w530
                tunnel: w529 -> [w537]
                tunnel: w528 -> [w535]
                stop <- w544 stop-if-true
                # "Status-Tacho-bit-M1 & M2"
                n178 = Build Array(w535, 114) -> (w542:i32[])
                n179 = call <vilib>:"i2c_sensors.vi"("Return Length"=2, "Bytes to Write"=w542, "NXT"=w537, "Port"=w538) -> ("Success?"=w534:bool, "Bytes read"=w539:u8[], "NXT"=w536:T2)  [unwired: 1 in]
                n180 = case shown="True" w534 {
                  tunnel: w539 -> [_ w564]
                  tunnel: [w556 w557] -> w549
                  tunnel: [w556 w559] -> w548
                  frame False {
                    w556 = u8 0
                  }
                  frame True {
                    n181 = Index Array(array=w564, index=0) -> (element=w560:u8)
                    n182 = Index Array(array=w564, index=1) -> (element=w558:u8)
                    n183 = And(x=w560, y=u8 8) -> (x .and. y?=w559:u8)
                    n184 = And(x=w558, y=u8 8) -> (x .and. y?=w557:u8)
                  }
                }
                n185 = Equal To 0?(x=w548) -> (x = 0?=w547:bool)
                n186 = Equal To 0?(x=w549) -> (x = 0?=w546:bool)
                n187 = And(x=w547, y=w546) -> (x .and. y?=w545:bool)
                n188 = case shown="True" w545 {
                  selector: w545 -> [w553 w555]
                  tunnel: w538 -> [_ _]
                  tunnel: [w553 w555] -> w544
                  tunnel: [w551 w554] -> w543
                  tunnel: w536 -> [w550 w554]
                  frame False {
                    n189 = call-poly <vilib>:"PolyWait.vi"("Time (100 msec)"=u16 50 ("Delay ms"), "NXT"=w550) -> ("NXT"=w551:T2)  [unwired: 2 in]
                  }
                  frame True {
                  }
                }
              }
            }
          }
        }
      }
    }
  }
  "NXT dup" <- w44
  n190 = Multiply(x=w70, y=0.0374) -> (x*y=w51:dbl)
  n191 = Index Array(array=w56, index=3) -> (element=w32:u8)
  n192 = Index Array(array=w56, index=2) -> (element=w31:u8)
  n193 = Index Array(array=w56, index=1) -> (element=w30:u8)
  n194 = Index Array(array=w56, index=0) -> (element=w29:u8)
  n195 = Index Array(array=w56, index=7) -> (element=w28:u8)
  n196 = Index Array(array=w56, index=6) -> (element=w27:u8)
  n197 = Index Array(array=w56, index=5) -> (element=w26:u8)
  n198 = Index Array(array=w56, index=4) -> (element=w25:u8)
  n199 = call <vilib>:"JoinH-L.vi"("low"=w31, "hi"=w32) -> ("(hi.lo)"=w24:u16)
  n200 = call <vilib>:"JoinH-L.vi"("low"=w29, "hi"=w30) -> ("(hi.lo)"=w23:u16)
  n201 = call <vilib>:"JoinH-L.vi"("low"=w27, "hi"=w28) -> ("(hi.lo)"=w21:u16)
  n202 = call <vilib>:"JoinH-L.vi"("low"=w25, "hi"=w26) -> ("(hi.lo)"=w20:u16)
  n203 = call <vilib>:"JoinH-L.vi"("low"=w23, "hi"=w24) -> ("(hi.lo)"=w22:u16)
  n204 = call <vilib>:"JoinH-L.vi"("low"=w20, "hi"=w21) -> ("(hi.lo)"=w19:u16)
  n205 = Bundle("millivolts"=w48, "(hi.lo)"=w22, "(hi.lo)"=w19, w51) -> ()  [unwired: 1 in, 1 out]
  n206 = Bundle(w47, "Out"=w46, w45) -> ()  [unwired: 1 in, 1 out]
